vi "Utility ASCII values.vi"() -> ()   [LabVIEW 2013]
panel:
  out "spreadsheet string":string
  out "unsigned byte array":u8[](array[numeric]) format="%.0x"
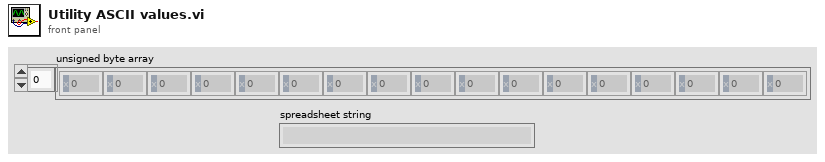
[diagram p1: front panel]
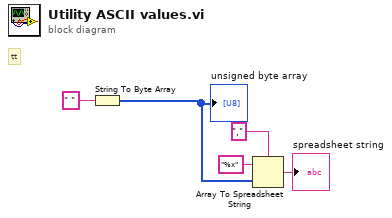
[diagram p0: block diagram]
diagram:
  # "tt"
  n1 = String To Byte Array(string=" ") -> (unsigned byte array=w4:u8[])
  "unsigned byte array" <- w4
  n2 = Array To Spreadsheet String(delimiter (Tab)=",", array=w4, 3:"%x" ("format string")) -> (spreadsheet string=→"spreadsheet string":string)
